vi "Read Sweep chunk.vi"(8 "error in (no error)":errorcluster, 11 "RUS Measurement in":refnum<class "RUS Measurement.lvclass">) -> (0 "error out":errorcluster, 2 "Sweep chunk":i32, 3 "RUS Measurement out":refnum<class "RUS Measurement.lvclass">)   [LabVIEW 2015, in "RUS Measurement.lvclass"]
uses:
  RUS Measurement.lvclass
  RUS Measurement.lvclass/RUS Measurement.ctl
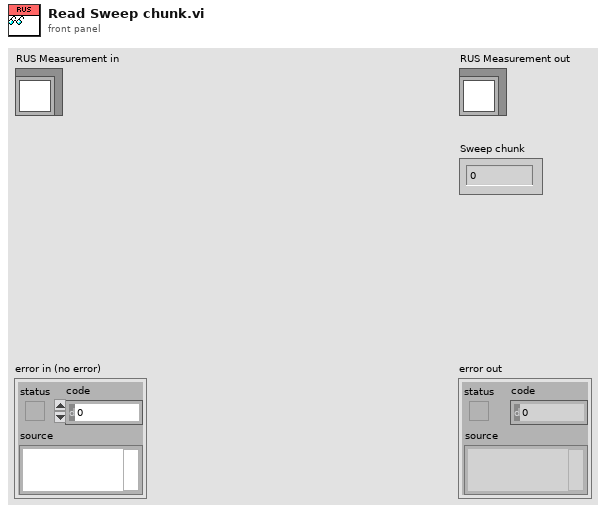
[diagram p1: front panel]
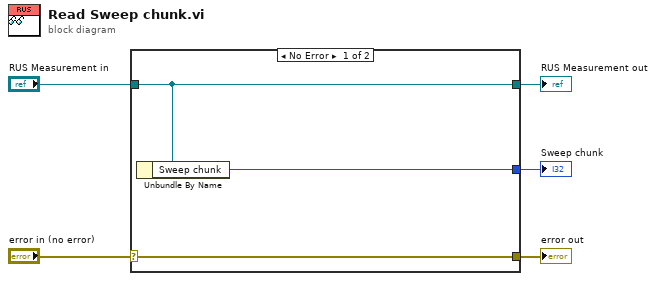
[diagram p0: block diagram]
diagram:
  n1 = case shown="No Error" "error in (no error)" {
    selector: "error in (no error)" -> [w8 w9]
    tunnel: [w8 w9] -> w4
    tunnel: [w7 w10] -> w2
    tunnel: "RUS Measurement in" -> [w7 w10]
    tunnel: [w6 _] -> w1
    frame No Error {
      n2 = Unbundle By Name(w7) -> ("Sweep chunk"=w6:i32)
    }
    frame Error {
    }
  }
  "error out" <- w4
  "RUS Measurement out" <- w2
  "Sweep chunk" <- w1
